vi "New License by Name.vi"(8 "error in (no error)":errorcluster, 11 "License Name":string) -> (0 "error out":errorcluster, 3 "CycloneDX License out":refnum<class "CycloneDX License.lvclass">)   [LabVIEW 2017, in "LabVIEW CycloneDX SBOM.lvlib" / "CycloneDX License.lvclass"]
doc: "Create a new license by name"
uses:
  CycloneDX License.lvclass
  C:/LabVIEW Working Directory/labview-cyclonedx-sbom/Source/CycloneDX/CycloneDX JSON/CycloneDX JSON.lvclass
  CycloneDX JSON/CycloneDX JSON.lvclass
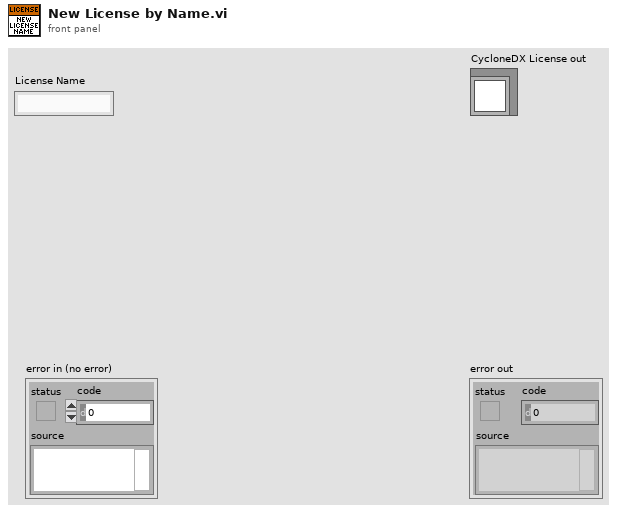
[diagram p1: front panel]
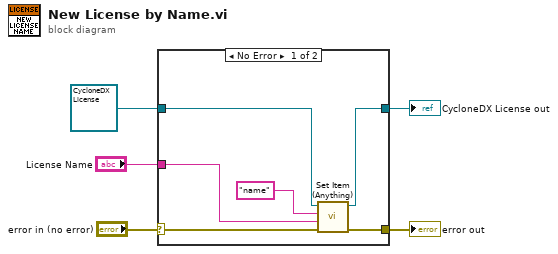
[diagram p0: block diagram]
diagram:
  n1 = case shown="No Error" "error in (no error)" {
    selector: "error in (no error)" -> [w9 w13]
    tunnel: [w8 w13] -> w4
    tunnel: [w10 w12] -> w2
    tunnel: refnum<class "CycloneDX License.lvclass"> refnum ("CycloneDX License in") -> [w11 w12]
    tunnel: "License Name" -> [w7 _]
    frame No Error {
      n2 = call "Set Item (Anything).vi"("error in (no error)"=w9, "Value"=w7, "Object (or Item) Path"="name", "CycloneDX SBOM in"=w11) -> ("error out"=w8:errorcluster, "CycloneDX SBOM out"=w10:refnum<class "CycloneDX License.lvclass">)  [unwired: 6 in]
    }
    frame Error {
    }
  }
  "error out" <- w4
  "CycloneDX License out" <- w2
